vi "Set Read Power.vi"(8 "error in (no error)":errorcluster, 9 "Power":u32=500 max=2700 step=10, 10 "Baud":u32=38400, 11 "COM Port":refnum<visa-resource-name>="COM4") -> (0 "error out":errorcluster, 1 "received str":string, 3 "Result":bool)   [LabVIEW 2018]
panel:
  out "Limmit":u32
  out "Size Array":u16
  out "Data Array":u8[](array[numeric]) format="%x"
  # "SET RX POWER"
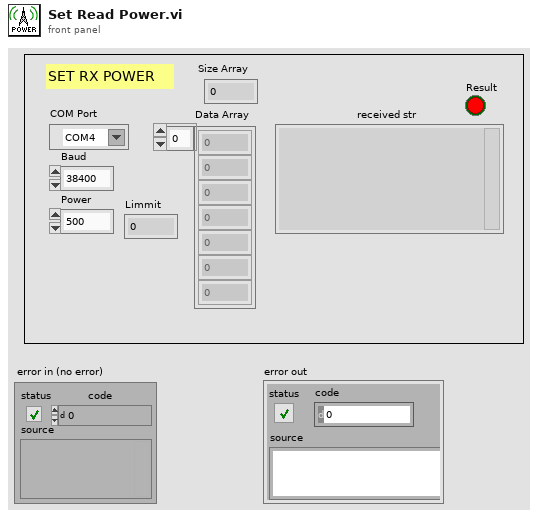
[diagram p1: front panel]
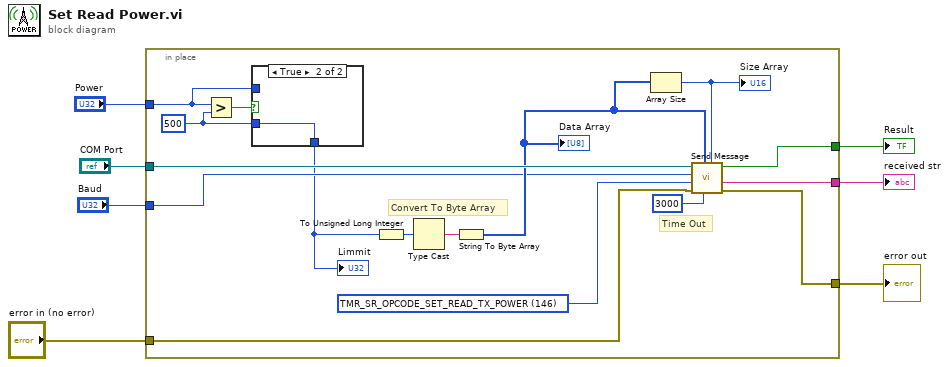
[diagram p0: block diagram]
diagram:
  n1 = in-place {
    in-place-border: "COM Port" -> [w22]
    in-place-border: [w19] -> w6
    in-place-border: [w18] -> w5
    in-place-border: "error in (no error)" -> [w15]
    in-place-border: "Baud" -> [w14]
    in-place-border: [w13] -> w2
    in-place-border: "Power" -> [w9]
    w10 = u32 500 ("y")
    w8 = u16 146 items=["TMR_SR_OPCODE_VERSION"=3, "TMR_SR_OPCODE_SET_BAUD_RATE"=6, "TMR_SR_OPCODE_READ_TAG_ID_SINGLE"=33, "TMR_SR_OPCODE_READ_TAG_ID_MULTIPLE"=34, "TMR_SR_OPCODE_WRITE_TAG_ID"=35, "TMR_SR_OPCODE_WRITE_TAG_DATA"=36, "TMR_SR_OPCODE_KILL_TAG"=38, "TMR_SR_OPCODE_READ_TAG_DATA"=40, "TMR_SR_OPCODE_CLEAR_TAG_ID_BUFFER"=42, "TMR_SR_OPCODE_MULTI_PROTOCOL_TAG_OP"=47, "TMR_SR_OPCODE_GET_READ_TX_POWER"=98, "TMR_SR_OPCODE_GET_WRITE_TX_POWER"=100, "TMR_SR_OPCODE_GET_POWER_MODE"=104, "TMR_SR_OPCODE_GET_READER_OPTIONAL_PARAMS"=106, "TMR_SR_OPCODE_GET_PROTOCOL_PARAM"=107, "TMR_SR_OPCODE_SET_ANTENNA_PORT"=145, "TMR_SR_OPCODE_SET_TAG_PROTOCOL"=147, "TMR_SR_OPCODE_SET_READ_TX_POWER"=146, "TMR_SR_OPCODE_SET_WRITE_TX_POWER"=148, "TMR_SR_OPCODE_SET_REGION"=151, "TMR_SR_OPCODE_SET_READER_OPTIONAL_PARAMS"=154, "TMR_SR_OPCODE_SET_PROTOCOL_PARAM"=155] ("Opcode Constant")
    # "Convert To Byte Array"
    # "Time Out"
    n2 = Greater?(x=w9, y=w10) -> (0:w12:bool)
    n3 = case shown="True" w12 {
      tunnel: [w24 w25] -> w11
      tunnel: w10 -> [_ w25]
      tunnel: w9 -> [w24 _]
      frame False {
      }
      frame True {
      }
    }
    "Limmit" <- w11
    n4 = To Unsigned Long Integer(number=w11) -> (unsigned 32bit integer=w23:u32)
    n5 = Type Cast(x=w23) -> (*(type *) &x=w17:string)  [unwired: 1 in]
    n6 = String To Byte Array(string=w17) -> (unsigned byte array=w16:u8[])
    "Data Array" <- w16
    n7 = Array Size(array=w16) -> (size(s)=w21:i32)
    "Size Array" <- w21
    n8 = call "Send Message.vi"("Size"=w21, "timeOut (ms)"=u32 3000, "Data"=w16, "error in (no error)"=w15, "Opcode"=w8, "Baud Rate"=w14, "COM Port"=w22) -> ("error out"=w18:errorcluster, "received str"=w13:string, "Result"=w19:bool)  [unwired: 1 in, 1 out]
  }
  "Result" <- w6
  "error out" <- w5
  "received str" <- w2
